vi "Host_Read_SimpleFPGA.vi"() -> ()   [LabVIEW 2018]
uses:
  <vilib>/rvi/interface/nirviOpenFPGA/nirviOpenFPGA.xnode
  <vilib>/rvi/interface/nirviReadWriteControl/nirviReadWriteControl.xnode
  <vilib>/rvi/interface/nirviCloseFPGA/nirviCloseFPGA.xnode
  <vilib>/rvi/interface/Simulation/niFpgaSimulationCallBeginRW.vi
  <vilib>/rvi/errors/niLvFpgaAdjustHostInterfaceError.vi
  ProjectFiles/FPGA Bitfiles/FPGALoopCountTest_2.lvbitx
  TestCode/FPGA_LoopCount_Test.vi
  <vilib>/FPGAPlugInAG/Dynamic/niLvFpga_Close_Dynamic.vi
panel:
  in  "WaitNoMore":bool
  out "error out 4":errorcluster
  out "HostLoopCount":i32
  out "DoneYet?":i32
  in  "stop":bool
  out "FPGALoopCount":i32
  out "error out 3":errorcluster
  out "error out 2":errorcluster
  out "error out":errorcluster
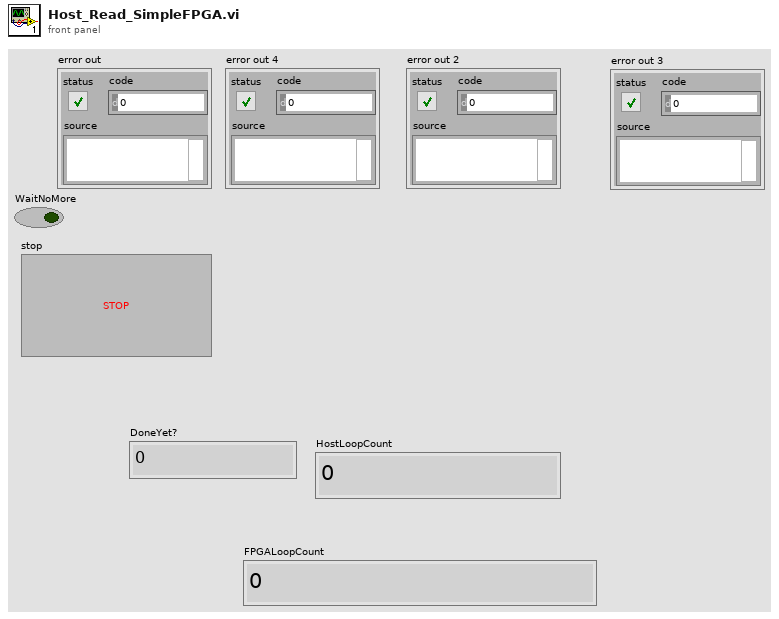
[diagram p1: front panel]
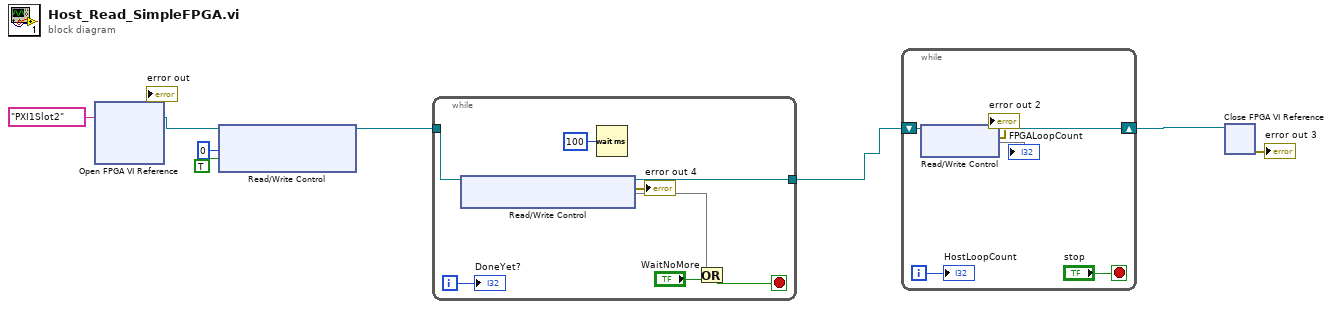
[diagram p0: block diagram]
diagram:
  n1 = xnode "Open FPGA VI Reference"("resource name"=tag "PXI1Slot2") -> ("FPGA VI Reference Out"=w4:refnum<k20>, "error out"=→"error out":errorcluster)  [unwired: 1 in]
  n2 = xnode "Read/Write Control"("FPGA VI Reference In"=w4, "Sample Clock Select"=u8 0, "Sample Clock Commit"=TRUE) -> ("FPGA VI Reference Out"=w3:refnum<k20>)  [unwired: 1 in, 1 out]
  n3 = while {
    tunnel: w3 -> [w17]
    tunnel: [w16] -> w5
    i -> [w13]
    stop <- w11 stop-if-true
    n4 = xnode "Read/Write Control"("FPGA VI Reference In"=w17) -> ("FPGA VI Reference Out"=w16:refnum<k20>, "error out"=→"error out 4":errorcluster, "IO Module\\Initialization Done"=w15)  [unwired: 1 in]
    n5 = Wait (ms)(milliseconds to wait=u32 100) -> ()  [unwired: 1 out]
    n6 = Or(x=w15, y="WaitNoMore") -> (x .or. y?=w11:bool)
    "DoneYet?" <- w13
  }
  n7 = while {
    shift-right: [w22] -> w8
    shift-left: w5 -> [w23]
    i -> [w18]
    stop <- "stop" stop-if-true
    n8 = xnode "Read/Write Control"("FPGA VI Reference In"=w23) -> ("FPGA VI Reference Out"=w22:refnum<k20>, "error out"=→"error out 2":errorcluster, "LoopCount"=→"FPGALoopCount")  [unwired: 1 in]
    "HostLoopCount" <- w18
  }
  n9 = xnode "Close FPGA VI Reference"("FPGA VI Reference In"=w8) -> ("error out"=→"error out 3":errorcluster)  [unwired: 1 in]
